vi "Config-Display-Graphics.vi"(0 "VISA session":refnum<visa-resource-name>, 1 "Y1 axis":T1={"name"="I3", "mode"=FALSE, "minimum"=0.0, "maximum"=0.1} {"maximum" format="%^.5e"; "minimum" format="%^.5e"}, 2 "data variable":bool, 5 "mode (X-Y1:0)":u16(ring), 7 "data variables":cluster{"variable1":string, "variable2":string}, 9 "X axis":T1={"name"="V3", "mode"=FALSE, "minimum"=0.0, "maximum"=1.0} {"maximum" format="%^.5e"; "minimum" format="%^.5e"}, 11 "error in (no error)":errorcluster, 12 "Y2 axis":T1={"name"="V1", "mode"=FALSE, "minimum"=0.0, "maximum"=3.0} {"maximum" format="%^.5e"; "minimum" format="%^.5e"}, 13 "grid":bool=TRUE) -> (4 "VISA resource name out":refnum<visa-resource-name>, 15 "error out":errorcluster)   [LabVIEW 2016, in "Agilent 415X Series.lvlib"]
doc: "This VI configures the axes and display status of grid and data variables. Executing this VI will automatically place the instrument in GRAPHICS display mode."
uses:
  Agilent 415X Series.lvlib
panel:
  # "This VI selects GRAPHICS display mode automatically."
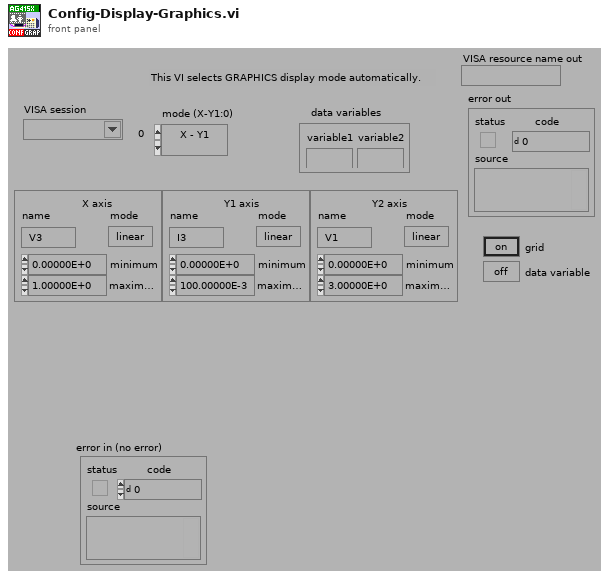
[diagram p1: front panel]
types:
  T1 = cluster{"name":string, "mode":bool, "minimum":dbl, "maximum":dbl}
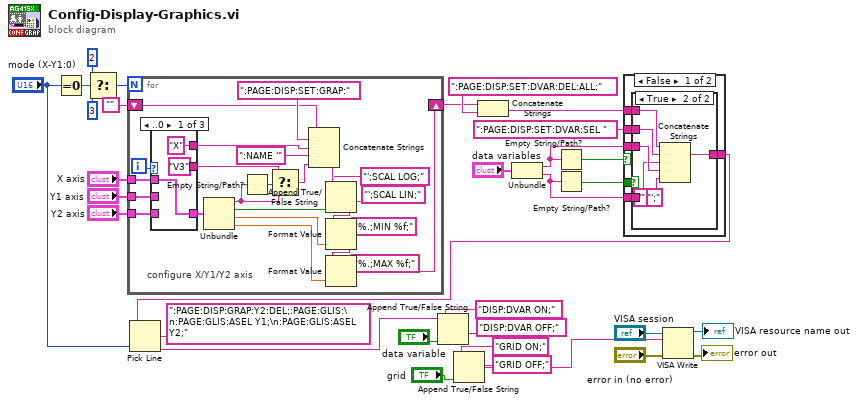
[diagram p0: block diagram]
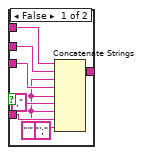
[diagram p2: hidden frame]
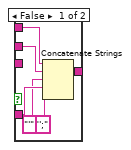
[diagram p4: hidden frame]
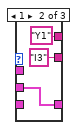
[diagram p5: hidden frame]
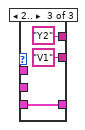
[diagram p6: hidden frame]
diagram:
  n1 = Equal To 0?(x="mode (X-Y1:0)") -> (x = 0?=w29:bool)
  n2 = Select(t=2, s=w29, f=3) -> (s? t:f=w30:i32)
  n3 = for {
    N: w30 -> [_]
    tunnel: "X axis" -> [w57]
    tunnel: "Y1 axis" -> [w56]
    tunnel: "Y2 axis" -> [w55]
    shift-right: [w37] -> w4
    shift-left: "" ("Empty String Constant") -> [w34]
    i -> [w54]
    # "configure X/Y1/Y2 axis"
    n4 = case shown="..0" w54 {
      tunnel: w57 -> [w60 _ _]
      tunnel: w56 -> [_ w63 _]
      tunnel: w55 -> [_ _ w66]
      tunnel: [w60 w63 w66] -> w52
      tunnel: ["X" "Y1" "Y2"] -> w36
      tunnel: ["V3" "I3" "V1"] -> w49
      frame ..0 {
      }
      frame 1 {
      }
      frame 2.. {
      }
    }
    n5 = Unbundle(w52) -> ("name"=w50:string, "mode"=w46:bool, "minimum"=w41:dbl, "maximum"=w40:dbl)
    n6 = Empty String/Path?(string/path=w50) -> (empty?=w51:bool)
    n7 = Select(t=w49, s=w51, f=w50) -> (s? t:f=w48:string)
    n8 = Concatenate Strings(w34, ":PAGE:DISP:SET:GRAP:", w36, ":NAME '", w48) -> (w47:string)
    n9 = Append True/False String(1:w46, 2:"';SCAL LIN;", 3:"';SCAL LOG;", 4:w47) -> (0:w43:string)
    n10 = Format Value(string ("")=w43, format string="%.;MIN %f;", value (0)=w41) -> (output string=w42:string)
    n11 = Format Value(string ("")=w42, format string="%.;MAX %f;", value (0)=w40) -> (output string=w37:string)
  }
  n12 = Concatenate Strings(w4, ":PAGE:DISP:SET:DVAR:DEL:ALL;") -> (w19:string)
  n13 = Unbundle("data variables") -> ("variable1"=w22:string, "variable2"=w21:string)
  n14 = Empty String/Path?(string/path=w22) -> (empty?=w24:bool)
  n15 = Empty String/Path?(string/path=w21) -> (empty?=w23:bool)
  n16 = case shown="False" w24 {
    tunnel: w23 -> [w72 w92]
    tunnel: w22 -> [w71 w91]
    tunnel: w21 -> [w70 w90]
    tunnel: w19 -> [w69 w89]
    tunnel: ":PAGE:DISP:SET:DVAR:SEL " -> [w68 w88]
    tunnel: [w67 w87] -> w18
    frame False {
      n17 = case shown="True" w72 {
        tunnel: w71 -> [w77 w83]
        tunnel: w70 -> [w74 _]
        tunnel: w69 -> [w80 w86]
        tunnel: w68 -> [w79 w85]
        tunnel: [w78 w84] -> w67
        frame False {
          w73 = "'"
          n18 = Concatenate Strings(w80, w79, w73, w77, w73, ",", w73, w74, "';") -> (w78:string)
        }
        frame True {
          n19 = Concatenate Strings(w86, w85, "'", w83, "';") -> (w84:string)
        }
      }
    }
    frame True {
      n20 = case shown="True" w92 {
        tunnel: w91 -> [_ _]
        tunnel: w90 -> [w95 _]
        tunnel: w89 -> [w98 w99]
        tunnel: w88 -> [w97 _]
        tunnel: [w96 w99] -> w87
        frame False {
          n21 = Concatenate Strings(w98, w97, "'", w95, "';") -> (w96:string)
        }
        frame True {
        }
      }
    }
  }
  n22 = Pick Line(string ("")=w18, multi-line string=":PAGE:DISP:GRAP:Y2:DEL;:PAGE:GLIS:\n:PAGE:GLIS:ASEL Y1;\n:PAGE:GLIS:ASEL Y2;", line index="mode (X-Y1:0)") -> (output string=w3:string)
  n23 = Append True/False String(1:"data variable", 2:"DISP:DVAR OFF;", 3:"DISP:DVAR ON;", 4:w3) -> (0:w9:string)
  n24 = Append True/False String(1:"grid", 2:"GRID OFF;", 3:"GRID ON;", 4:w9) -> (0:w2:string)
  n25 = VISA Write(VISA resource name="VISA session", write buffer=w2, error in (no error)="error in (no error)") -> (VISA resource name out=→"VISA resource name out":refnum<visa-resource-name>, error out=→"error out":errorcluster)  [unwired: 1 out]
